vi "HeinzingerAndKepcoTest.vi"() -> ()   [LabVIEW 2014]
uses:
  Controls/DacState.ctl
  Controls/heinzingerSelect.ctl
  <vilib>/rvi/Emulation/niFpgaGetClockAttributes.vi
  <vilib>/rvi/Emulation/niFpgaSctlEmulationGetInTimedLoop.vi
  <vilib>/rvi/Emulation/niFpgaEmulationReportErrorSimple.vi
  DAC/Code/FPGA SPI_Globals.vi
  HeinzingerControl/heinzingerControlGlobals.vi
  <vilib>/rvi/Emulation/niFpgaCriticalErrorInLSC.vi
panel:
  out "postAccOffsetVoltState":T1
  in  "postAccOffsetVoltControl":T1
  out "DacState":T2
  out "actDACRegister":u32=1572792 caption="actRegister" format="%024b"
  in  "setDACRegister":u32=1048576 format="%024b"
  in  "DacStateCmdByHost":T2
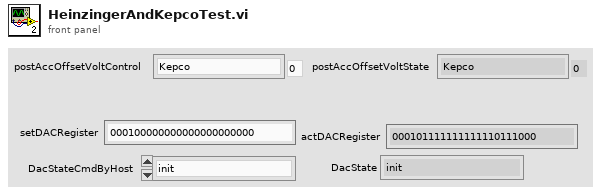
[diagram p1: front panel]
types:
  T1 = typedef "heinzingerSelect.ctl" = enum8{"Kepco", "Heinzinger0", "Heinzinger1", "Heinzinger2", "loading"}
  T2 = typedef "DacState.ctl" = enum16{"init", "idle", "setVolt", "error"}
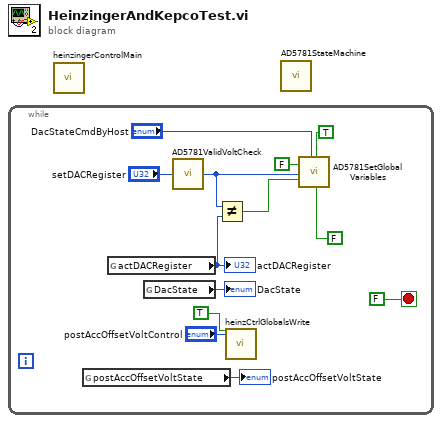
[diagram p0: block diagram]
diagram:
  n1 = while {
    stop <- FALSE stop-if-true
    n2 = global read "heinzingerControlGlobals.vi" "postAccOffsetVoltState"() -> (→"postAccOffsetVoltState":T1)
    n3 = global read "FPGA SPI_Globals.vi" "actDACRegister"() -> (w9:u32)
    "actDACRegister" <- w9
    n4 = global read "FPGA SPI_Globals.vi" "DacState"() -> (→"DacState":T2)
    n5 = call "AD5781ValidVoltCheck.vi"("U32"="setDACRegister") -> ("coerced(x)"=w7:u32)  [unwired: 4 in]
    n6 = Not Equal?(x=w7, y=w9) -> (x != y?=w8:bool)
    n7 = call "heinzCtrlGlobalsWrite.vi"("w_postAccOffsetVoltControl"=TRUE, "postAccOffsetVoltControl"="postAccOffsetVoltControl") -> ()  [unwired: 26 in]
    n8 = call "AD5781SetGlobalVariables.vi"("write actDACRegister"=FALSE, "setDACRegister"=w7, "write setDACRegister"=w8, "DacStateCmdByHost"="DacStateCmdByHost", "write DacStateCmdByHost"=TRUE, "write DacState"=FALSE) -> ()  [unwired: 14 in]
  }
  n9 = call "heinzingerControlMain.vi"() -> ()  [unwired: 3 in]
  n10 = call "AD5781StateMachine.vi"() -> ()  [unwired: 12 in]
